vi "main.vi"(8 "error in (no error)":errorcluster, 11 "context out":refnum<class "zmq_context.lvclass">) -> (0 "error out":errorcluster)   [LabVIEW 2020, in "ui-testing.lvlib"]
doc: "Main implementation of the User Interface testing daemon.\ncopyright: Thomas Zilliox©"
uses:
  ui-testing.lvlib
  <vilib>/addons/zeromq/zmq_context.lvclass
  <vilib>/addons/zeromq/socket_type.ctl
  <vilib>/addons/zeromq/zeromq.lvlib
  <vilib>/addons/zeromq/zmq_socket.lvclass
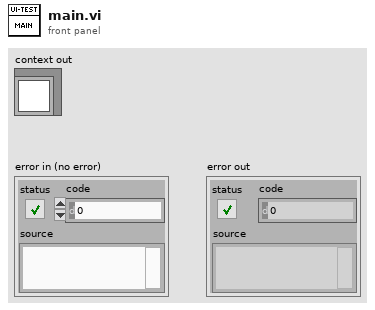
[diagram p1: front panel]
types:
  T1 = typedef "zeromq.lvlib/socket_type.ctl" = enum8{"ZMQ_PAIR", "ZMQ_PUB", "ZMQ_SUB", "ZMQ_REQ", "ZMQ_REP", "ZMQ_DEALER", "ZMQ_ROUTER", "ZMQ_PULL", "ZMQ_PUSH", "ZMQ_XPUB", "ZMQ_XSUB", "ZMQ_STREAM", "ZMQ_SERVER", "ZMQ_CLIENT", "ZMQ_RADIO", "ZMQ_DISH", "ZMQ_GATHER", "ZMQ_SCATTER", "ZMQ_DGRAM"}
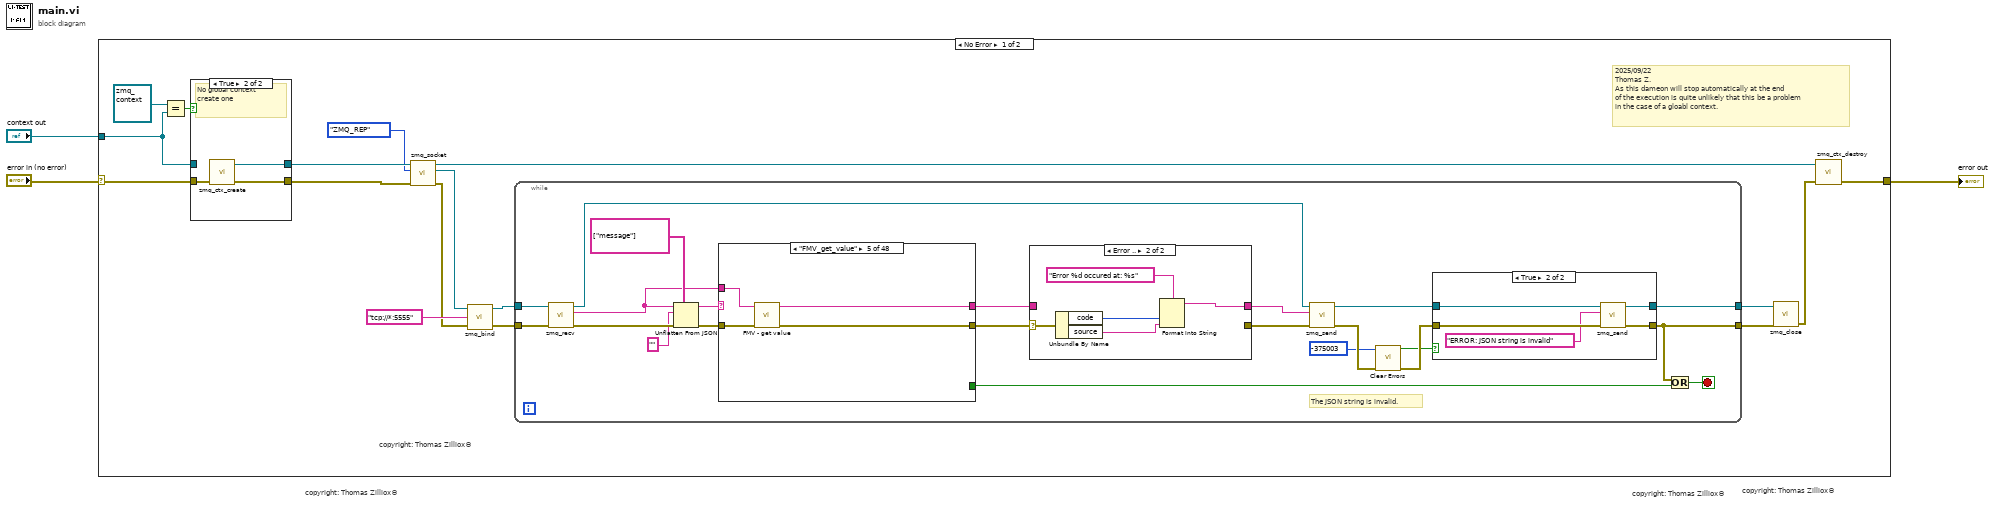
[diagram p0: block diagram]
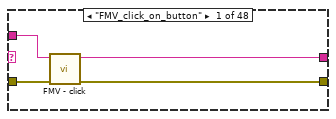
[diagram p5: hidden frame]
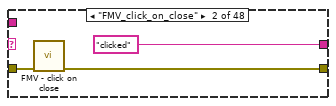
[diagram p6: hidden frame]
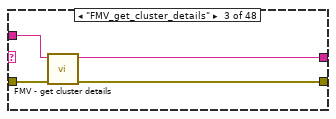
[diagram p7: hidden frame]
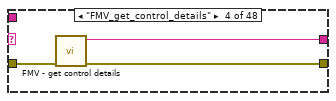
[diagram p8: hidden frame]
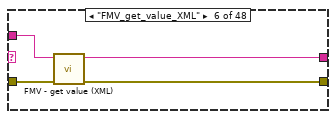
[diagram p9: hidden frame]
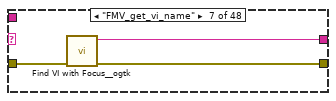
[diagram p10: hidden frame]
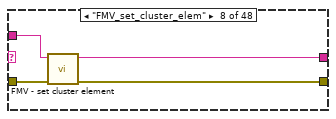
[diagram p11: hidden frame]
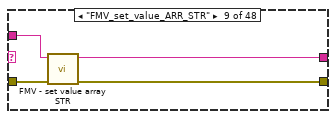
[diagram p12: hidden frame]
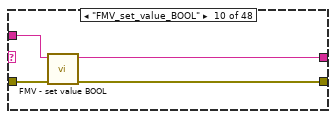
[diagram p13: hidden frame]
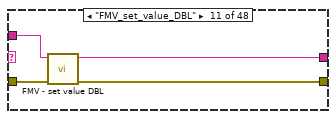
[diagram p14: hidden frame]
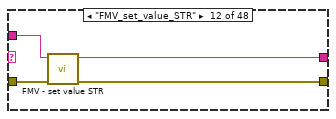
[diagram p15: hidden frame]
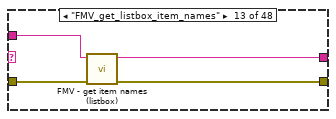
[diagram p16: hidden frame]
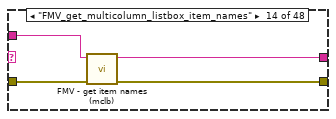
[diagram p17: hidden frame]
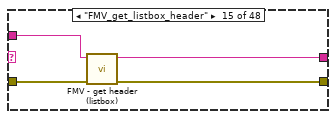
[diagram p18: hidden frame]
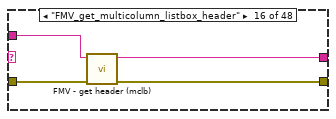
[diagram p19: hidden frame]
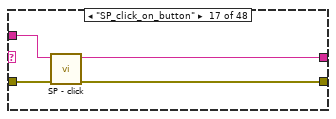
[diagram p20: hidden frame]
diagram:
  # "copyright: Thomas Zilliox©"
  # "copyright: Thomas Zilliox©"
  # "copyright: Thomas Zilliox©"
  n1 = case shown="No Error" "error in (no error)" {
    selector: "error in (no error)" -> [w8 w248]
    tunnel: [w7 w248] -> w2
    tunnel: "context out" -> [w4 _]
    frame No Error {
      # "2025/09/22\nThomas Z.\nAs this dameon will stop automatically at the end\nof the execution is quite unlikely that this be a problem\nin the case of a gloabl context."
      # "copyright: Thomas Zilliox©"
      n2 = Equal?(x=refnum<class "zmq_context.lvclass"> refnum ("context out"), y=w4) -> (x = y?=w5:bool)
      n3 = case shown="True" w5 {
        tunnel: [w21 w25] -> w20
        tunnel: [w22 w24] -> w19
        tunnel: w8 -> [w22 w23]
        tunnel: w4 -> [w21 _]
        frame False {
          # "Use the context of the application"
        }
        frame True {
          # "No global context\ncreate one"
          n4 = call <vilib>:"zmq_ctx_create.vi"("error in"=w23) -> ("error out"=w24:errorcluster, "context out"=w25:refnum<class "zmq_context.lvclass">)  [unwired: 3 in]
        }
      }
      n5 = call <vilib>:"zmq_socket.vi"("error in"=w19, "socket type"=socket_type."ZMQ_REP", "context in"=w20) -> ("error out"=w14:errorcluster, "socket out"=w16:refnum<class "zmq_socket.lvclass">, "context out"=w17:refnum<class "zmq_context.lvclass">)  [unwired: 2 in]
      n6 = call <vilib>:"zmq_bind.vi"("error in"=w14, "endpoint"="tcp://*:5555", "socket in"=w16) -> ("error out"=w12:errorcluster, "socket out"=w13:refnum<class "zmq_socket.lvclass">)  [unwired: 1 in]
      n7 = while {
        tunnel: w13 -> [w47]
        tunnel: w12 -> [w46]
        tunnel: [w33] -> w11
        tunnel: [w31] -> w10
        stop <- w43 stop-if-true
        # "The JSON string is invalid."
        n8 = call <vilib>:"zmq_recv.vi"("error in"=w46, "socket in"=w47) -> ("error out"=w41:errorcluster, "data"=w36:string, "socket out"=w45:refnum<class "zmq_socket.lvclass">)  [unwired: 3 in, 2 out]
        n9 = Unflatten From JSON(path=string[] ["message"], JSON string=w36, type and defaults="", error in (no error)=w41) -> (value=w38:string, error out=w40:errorcluster)  [unwired: 3 in]
        n10 = case shown="\"FMV_get_value\"" w38 {
          tunnel: [w63 w67 w69 w73 w76 w81 w85 w87 w91 w95 w99 w103 w109 w113 w117 w121 w124 w127 w132 w135 w140 w144 w148 w152 w156 w161 w163 w167 w171 w175 w179 w184 w188 w192 w197 w200 w204 w208 w211 w216 w220 w224 w228 w232 w235 w240 w245 w247] -> w29
          tunnel: w40 -> [w64 w68 w72 w75 w78 w82 w86 w90 w94 w98 w102 w106 w110 w114 w118 w122 w125 w130 w134 w137 w141 w145 w149 w153 w157 w162 w166 w169 w173 w177 w181 w185 w190 w193 w198 w201 w205 w209 w214 w217 w221 w225 w229 w233 w238 w241 w245 w247]
          tunnel: [_ _ _ _ _ _ _ _ _ _ _ _ _ _ _ _ _ _ _ _ _ _ _ _ _ _ _ _ _ _ _ _ _ _ _ _ _ _ _ _ _ _ _ _ _ _ TRUE _] -> w42
          tunnel: [w62 "clicked" ("VI Name") w70 w74 w77 w80 w84 w88 w92 w96 w100 w104 w107 w111 w115 w119 w123 w128 w133 w136 w139 w143 w147 w151 w155 w160 w164 w168 w172 w176 w180 w183 w189 w191 w196 w199 w203 w207 w212 w215 w219 w223 w227 w231 w236 w239 "ciao!" ("data") "Undefinied" ("data")] -> w27
          tunnel: w36 -> [w65 _ w71 _ w79 w83 _ w89 w93 w97 w101 w105 w108 w112 w116 w120 w126 w129 w131 w138 w142 w146 w150 w154 w158 w159 w165 w170 w174 w178 w182 w186 w187 w194 w195 w202 w206 w210 w213 w218 w222 w226 w230 w234 w237 w242 _ _]
          frame "FMV_click_on_button" {
            n11 = call "FMV - click.vi"("error in (no error)"=w64, "JSON string"=w65) -> ("error out"=w63:errorcluster, "value"=w62:string)  [unwired: 8 in]
          }
          frame "FMV_click_on_close" {
            n12 = call "FMV - click on close.vi"("error in (no error)"=w68) -> ("error out"=w67:errorcluster)  [unwired: 10 in]
          }
          frame "FMV_get_cluster_details" {
            n13 = call "FMV - get cluster details.vi"("error in (no error)"=w72, "JSON string"=w71) -> ("error out"=w69:errorcluster, "value"=w70:string)  [unwired: 8 in]
          }
          frame "FMV_get_control_details" {
            n14 = call "FMV - get control details.vi"("error in (no error)"=w75) -> ("error out"=w73:errorcluster, "Control details"=w74:string)  [unwired: 9 in]
          }
          frame "FMV_get_value" {
            n15 = call "FMV - get value.vi"("error in (no error)"=w78, "JSON string"=w79) -> ("error out"=w76:errorcluster, "value"=w77:string)  [unwired: 8 in]
          }
          frame "FMV_get_value_XML" {
            n16 = call "FMV - get value (XML).vi"("error in (no error)"=w82, "JSON string"=w83) -> ("error out"=w81:errorcluster, "value"=w80:string)  [unwired: 8 in]
          }
          frame "FMV_get_vi_name" {
            n17 = call <userlib>:"Find VI with Focus__ogtk.vi"("error in"=w86) -> ("error out"=w85:errorcluster, "VI Name"=w84:string)  [unwired: 6 in, 3 out]
          }
          frame "FMV_set_cluster_elem" {
            n18 = call "FMV - set cluster element.vi"("error in (no error)"=w90, "JSON string"=w89) -> ("error out"=w87:errorcluster, "value"=w88:string)  [unwired: 8 in]
          }
          frame "FMV_set_value_ARR_STR" {
            n19 = call "FMV - set value array STR.vi"("error in (no error)"=w94, "JSON string"=w93) -> ("error out"=w91:errorcluster, "value"=w92:string)  [unwired: 8 in]
          }
          frame "FMV_set_value_BOOL" {
            n20 = call "FMV - set value BOOL.vi"("error in (no error)"=w98, "JSON string"=w97) -> ("error out"=w95:errorcluster, "value"=w96:string)  [unwired: 8 in]
          }
          frame "FMV_set_value_DBL" {
            n21 = call "FMV - set value DBL.vi"("error in (no error)"=w102, "JSON string"=w101) -> ("error out"=w99:errorcluster, "value"=w100:string)  [unwired: 8 in]
          }
          frame "FMV_set_value_STR" {
            n22 = call "FMV - set value STR.vi"("error in (no error)"=w106, "JSON string"=w105) -> ("error out"=w103:errorcluster, "value"=w104:string)  [unwired: 8 in]
          }
          frame "FMV_get_listbox_item_names" {
            n23 = call "FMV - get item names (listbox).vi"("error in (no error)"=w110, "JSON string"=w108) -> ("error out"=w109:errorcluster, "value"=w107:string)  [unwired: 8 in]
          }
          frame "FMV_get_multicolumn_listbox_item_names" {
            n24 = call "FMV - get item names (mclb).vi"("error in (no error)"=w114, "JSON string"=w112) -> ("error out"=w113:errorcluster, "value"=w111:string)  [unwired: 8 in]
          }
          frame "FMV_get_listbox_header" {
            n25 = call "FMV - get header (listbox).vi"("error in (no error)"=w118, "JSON string"=w116) -> ("error out"=w117:errorcluster, "value"=w115:string)  [unwired: 8 in]
          }
          frame "FMV_get_multicolumn_listbox_header" {
            n26 = call "FMV - get header (mclb).vi"("error in (no error)"=w122, "JSON string"=w120) -> ("error out"=w121:errorcluster, "value"=w119:string)  [unwired: 8 in]
          }
          frame "SP_click_on_button" {
            n27 = call "SP - click.vi"("error in (no error)"=w125, "JSON string"=w126) -> ("error out"=w124:errorcluster, "value"=w123:string)  [unwired: 8 in]
          }
          frame "SP_get_cluster_details" {
            n28 = call "SP - get cluster details.vi"("error in (no error)"=w130, "JSON string"=w129) -> ("error out"=w127:errorcluster, "value"=w128:string)  [unwired: 8 in]
          }
          frame "SP_get_control_details" {
            n29 = call "SP - get control details.vi"("error in (no error)"=w134, "JSON string"=w131) -> ("error out"=w132:errorcluster, "value"=w133:string)  [unwired: 8 in]
          }
          frame "SP_get_value" {
            n30 = call "SP - get value.vi"("error in (no error)"=w137, "JSON string"=w138) -> ("error out"=w135:errorcluster, "value"=w136:string)  [unwired: 8 in]
          }
          frame "SP_get_value_XML" {
            n31 = call "SP - get value (XML).vi"("error in (no error)"=w141, "JSON string"=w142) -> ("error out"=w140:errorcluster, "value"=w139:string)  [unwired: 8 in]
          }
          frame "SP_get_listbox_item_names" {
            n32 = call "SP - get item names (listbox).vi"("error in (no error)"=w145, "JSON string"=w146) -> ("error out"=w144:errorcluster, "value"=w143:string)  [unwired: 8 in]
          }
          frame "SP_get_multicolumn_listbox_item_names" {
            n33 = call "SP - get item names (mclb).vi"("error in (no error)"=w149, "JSON string"=w150) -> ("error out"=w148:errorcluster, "value"=w147:string)  [unwired: 8 in]
          }
          frame "SP_get_listbox_header" {
            n34 = call "SP - get header (listbox).vi"("error in (no error)"=w153, "JSON string"=w154) -> ("error out"=w152:errorcluster, "value"=w151:string)  [unwired: 8 in]
          }
          frame "SP_get_multicolumn_listbox_header" {
            n35 = call "SP - get header (mclb).vi"("error in (no error)"=w157, "JSON string"=w158) -> ("error out"=w156:errorcluster, "value"=w155:string)  [unwired: 8 in]
          }
          frame "SP_get_vi_name" {
            n36 = call "SP - Get current VI name.vi"("error in (no error)"=w162, "JSON string"=w159) -> ("error out"=w161:errorcluster, "value"=w160:string)  [unwired: 8 in]
          }
          frame "SP_set_cluster_elem" {
            n37 = call "SP - set cluster element.vi"("error in (no error)"=w166, "JSON string"=w165) -> ("error out"=w163:errorcluster, "value"=w164:string)  [unwired: 8 in]
          }
          frame "SP_set_value_ARR_STR" {
            n38 = call "SP - set value array STR.vi"("error in (no error)"=w169, "JSON string"=w170) -> ("error out"=w167:errorcluster, "value"=w168:string)  [unwired: 8 in]
          }
          frame "SP_set_value_BOOL" {
            n39 = call "SP - set value BOOL.vi"("error in (no error)"=w173, "JSON string"=w174) -> ("error out"=w171:errorcluster, "value"=w172:string)  [unwired: 8 in]
          }
          frame "SP_set_value_DBL" {
            n40 = call "SP - set value DBL.vi"("error in (no error)"=w177, "JSON string"=w178) -> ("error out"=w175:errorcluster, "value"=w176:string)  [unwired: 8 in]
          }
          frame "SP_set_value_STR" {
            n41 = call "SP - set value STR.vi"("error in (no error)"=w181, "JSON string"=w182) -> ("error out"=w179:errorcluster, "value"=w180:string)  [unwired: 8 in]
          }
          frame "SP_SP_click_on_button" {
            n42 = call "SSP - click.vi"("error in (no error)"=w185, "JSON string"=w186) -> ("error out"=w184:errorcluster, "value"=w183:string)  [unwired: 8 in]
          }
          frame "SP_SP_get_control_details" {
            n43 = call "SSP - get control details.vi"("error in (no error)"=w190, "JSON string"=w187) -> ("error out"=w188:errorcluster, "value"=w189:string)  [unwired: 8 in]
          }
          frame "SP_SP_get_value" {
            n44 = call "SSP - get value.vi"("error in (no error)"=w193, "JSON string"=w194) -> ("error out"=w192:errorcluster, "value"=w191:string)  [unwired: 8 in]
          }
          frame "SP_SP_get_vi_name" {
            n45 = call "SSP - Get current VI name.vi"("error in (no error)"=w198, "JSON string"=w195) -> ("error out"=w197:errorcluster, "value"=w196:string)  [unwired: 8 in]
          }
          frame "SP_SP_set_value_ARR_STR" {
            n46 = call "SSP - set value array STR.vi"("error in (no error)"=w201, "JSON string"=w202) -> ("error out"=w200:errorcluster, "value"=w199:string)  [unwired: 8 in]
          }
          frame "SP_SP_set_value_DBL" {
            n47 = call "SSP - set value DBL.vi"("error in (no error)"=w205, "JSON string"=w206) -> ("error out"=w204:errorcluster, "value"=w203:string)  [unwired: 8 in]
          }
          frame "SP_SP_set_value_STR" {
            n48 = call "SSP - set value STR.vi"("error in (no error)"=w209, "JSON string"=w210) -> ("error out"=w208:errorcluster, "value"=w207:string)  [unwired: 8 in]
          }
          frame "SSP_get_cluster_details" {
            n49 = call "SSP - get cluster detailst.vi"("error in (no error)"=w214, "JSON string"=w213) -> ("error out"=w211:errorcluster, "value"=w212:string)  [unwired: 8 in]
          }
          frame "SSP_get_value_XML" {
            n50 = call "SSP - get value (XML).vi"("error in (no error)"=w217, "JSON string"=w218) -> ("error out"=w216:errorcluster, "value"=w215:string)  [unwired: 8 in]
          }
          frame "SSP_get_listbox_item_names" {
            n51 = call "SSP - get item names (listbox).vi"("error in (no error)"=w221, "JSON string"=w222) -> ("error out"=w220:errorcluster, "value"=w219:string)  [unwired: 8 in]
          }
          frame "SSP_get_multicolumn_listbox_item_names" {
            n52 = call "SSP - get item names (mclb).vi"("error in (no error)"=w225, "JSON string"=w226) -> ("error out"=w224:errorcluster, "value"=w223:string)  [unwired: 8 in]
          }
          frame "SSP_get_listbox_header" {
            n53 = call "SSP - get header (listbox).vi"("error in (no error)"=w229, "JSON string"=w230) -> ("error out"=w228:errorcluster, "value"=w227:string)  [unwired: 8 in]
          }
          frame "SSP_get_multicolumn_listbox_header" {
            n54 = call "SSP - get header (mclb).vi"("error in (no error)"=w233, "JSON string"=w234) -> ("error out"=w232:errorcluster, "value"=w231:string)  [unwired: 8 in]
          }
          frame "SSP_set_cluster_elem" {
            n55 = call "SSP - set cluster element.vi"("error in (no error)"=w238, "JSON string"=w237) -> ("error out"=w235:errorcluster, "value"=w236:string)  [unwired: 8 in]
          }
          frame "SSP_set_value_BOOL" {
            n56 = call "SSP - set value BOOL.vi"("error in (no error)"=w241, "JSON string"=w242) -> ("error out"=w240:errorcluster, "value"=w239:string)  [unwired: 8 in]
          }
          frame "stop" {
          }
          frame Default {
          }
        }
        n57 = case shown="Error .." w29 {
          selector: w29 -> [w48 w54]
          tunnel: [w49 w50] -> w28
          tunnel: w27 -> [w49 _]
          tunnel: [w48 _] -> w26
          frame No Error {
          }
          frame Error {
            n58 = Unbundle By Name(w54) -> ("code"=w52:i32, "source"=w51:string)
            n59 = Format Into String(format string="Error %d occured at: %s", w52, w51) -> (resulting string=w50:string)  [unwired: 2 in, 1 out]
          }
        }
        n60 = call <vilib>:"zmq_send.vi"("error in"=w26, "data"=w28, "socket in"=w45) -> ("error out"=w44:errorcluster, "socket out"=w34:refnum<class "zmq_socket.lvclass">)  [unwired: 4 in]
        n61 = call <vilib>:"Clear Errors.vi"("error in (no error)"=w44, "specific error code to clear (0: all)"=-375003) -> ("error out"=w32:errorcluster, "specific error cleared?"=w30:bool)  [unwired: 4 in]
        n62 = case shown="True" w30 {
          tunnel: w34 -> [w56 w61]
          tunnel: [w56 w60] -> w33
          tunnel: w32 -> [w55 w59]
          tunnel: [w55 w58] -> w31
          frame False {
          }
          frame True {
            n63 = call <vilib>:"zmq_send.vi"("error in"=w59, "data"="ERROR: JSON string is invalid", "socket in"=w61) -> ("error out"=w58:errorcluster, "socket out"=w60:refnum<class "zmq_socket.lvclass">)  [unwired: 4 in]
          }
        }
        n64 = Or(x=w31, y=w42) -> (x .or. y?=w43:bool)
      }
      n65 = call <vilib>:"zmq_close.vi"("error in"=w10, "socket"=w11) -> ("error out"=w9:errorcluster)  [unwired: 3 in]
      n66 = call <vilib>:"zmq_ctx_destroy.vi"("error in"=w9, "context in"=w17) -> ("error out"=w7:errorcluster)  [unwired: 3 in]
    }
    frame Error {
      # "copyright: Thomas Zilliox©"
    }
  }
  "error out" <- w2
